vi "Untitled 3.vi"   [LabVIEW 2017]
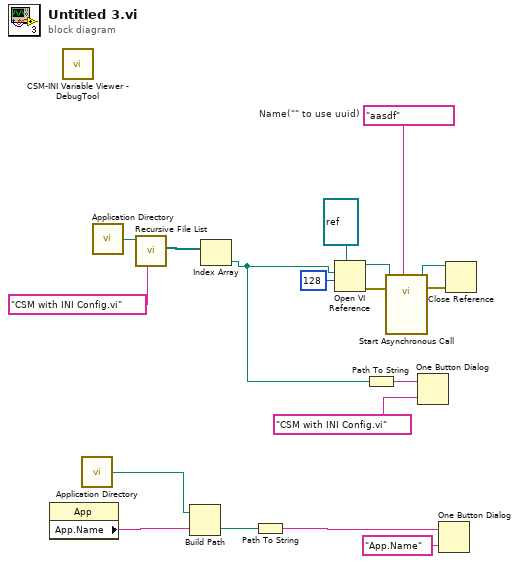
[diagram p0: block diagram]
diagram:
  w15 = "aasdf"  # Name("" to use uuid)
  n1 = property class="App"() -> ("App.Name"=w6:string)  [unwired: 2 in, 2 out]
  n2 = call "CSM-INI Variable Viewer - DebugTool.vi"() -> ()  [unwired: 12 in]
  n3 = call <vilib>:"Application Directory.vi"() -> ("Application Directory"=w2:path)
  n4 = call <vilib>:"Application Directory.vi"() -> ("Application Directory"=w10:path)
  n5 = call <vilib>:"Recursive File List.vi"("pattern"="CSM with INI Config.vi", "Folder Path"=w10) -> ("All Files in Dir"=w8:path[])  [unwired: 5 in, 4 out]
  n6 = Build Path(base path=w2, name or relative path=w6) -> (appended path=w3:path)
  n7 = Index Array(array=w8) -> (element=w7:path)  [unwired: 1 in]
  n8 = Path To String(path=w3) -> (string=w1:string)
  n9 = Open VI Reference(type specifier VI Refnum (for type only)=refnum<vi> refnum, vi path=w7, options=128) -> (vi reference=w11:refnum<vi>, error out=w14:errorcluster)  [unwired: 3 in]
  n10 = Path To String(path=w7) -> (string=w13:string)
  n11 = call-by-ref "Start Asynchronous Call"(reference=w11, error in=w14, "Name(\"\" to use uuid)"=w15) -> (reference out=w17:refnum<vi>, error out=w16:errorcluster)  [unwired: 11 in]
  n12 = One Button Dialog(message=w13, button name ("OK")="CSM with INI Config.vi") -> ()  [unwired: 1 out]
  n13 = One Button Dialog(message=w1, button name ("OK")="App.Name") -> ()  [unwired: 1 out]
  n14 = Close Reference(reference=w17, error in (no error)=w16) -> ()  [unwired: 1 out]
